vi "FinishServo.vi"   [LabVIEW 2015]
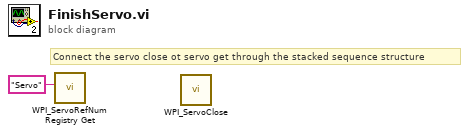
[diagram p0: block diagram]
diagram:
  # "Connect the servo close ot servo get through the stacked sequence structure"
  n1 = call <vilib>:"WPI_ServoRefNum Registry Get.vi"("refnum name"="Servo") -> ()  [unwired: 9 in, 2 out]
  n2 = call <vilib>:"WPI_ServoClose.vi"() -> ()  [unwired: 11 in, 1 out]
